vi "02 LinkTest.vi"(8 "error in (no error)":errorcluster caption="错误输入（无错误）", 10 "串口配置":T1={"VISA串口名称"="", "波特率"=9600, "停止位"=10, "流控制"=0, "数据位"=8, "奇偶校验"=enum."None", "超时"=2000, "启用终止符？"=FALSE, "终止符"=10} {"终止符" format="%.0x"; "数据位" min=5 max=8 step=1; "流控制" items=["无", "XON/XOFF", "RTS/CTS", "XON/XOFF & RTS/CTS", "DTR/DSR", "XON/XOFF & DTR/DSR"]; "停止位" items=["1.0"=10, "1.5"=15, "2.0"=20]; "波特率" items=["9600"=9600, "115200"=15]}, 11 "SerialClass 输入":refnum<class "SerialClass.lvclass">) -> (0 "error out":errorcluster caption="错误输出", 1 "串口已配置":T1={"VISA串口名称"="", "波特率"=9600, "停止位"=10, "流控制"=0, "数据位"=8, "奇偶校验"=enum."None", "超时"=2000, "启用终止符？"=FALSE, "终止符"=10} {"终止符" format="%.0x"; "数据位" min=5 max=8 step=1; "流控制" items=["无", "XON/XOFF", "RTS/CTS", "XON/XOFF & RTS/CTS", "DTR/DSR", "XON/XOFF & DTR/DSR"]; "停止位" items=["1.0"=10, "1.5"=15, "2.0"=20]; "波特率" items=["9600"=9600, "115200"=15]}, 2 "成功？":bool, 3 "SerialClass 输出":refnum<class "SerialClass.lvclass">)   [LabVIEW 2019, in "SerialClass.lvclass"]
uses:
  SerialClass.lvclass
  00 Ctl/SerialData.ctl
  <vilib>/Instr/_visa.llb/VISA Configure Serial Port (Instr).vi
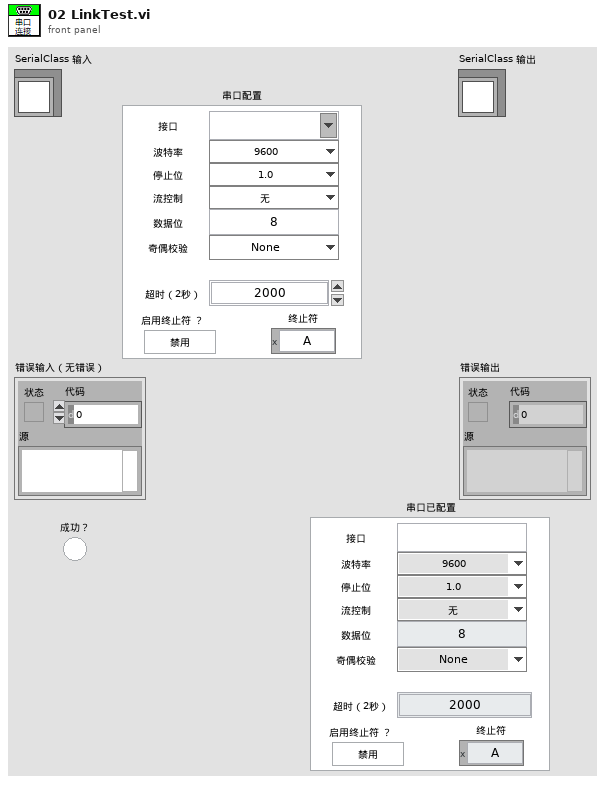
[diagram p1: front panel]
types:
  T1 = typedef "SerialData.ctl" = cluster{"VISA串口名称":refnum<visa-resource-name>, "波特率":u32, "停止位":u16, "流控制":u16, "数据位":u16, "奇偶校验":enum16{"None", "Odd", "Even", "Mark", "Space"}, "超时":u32, "启用终止符？":bool, "终止符":u8}
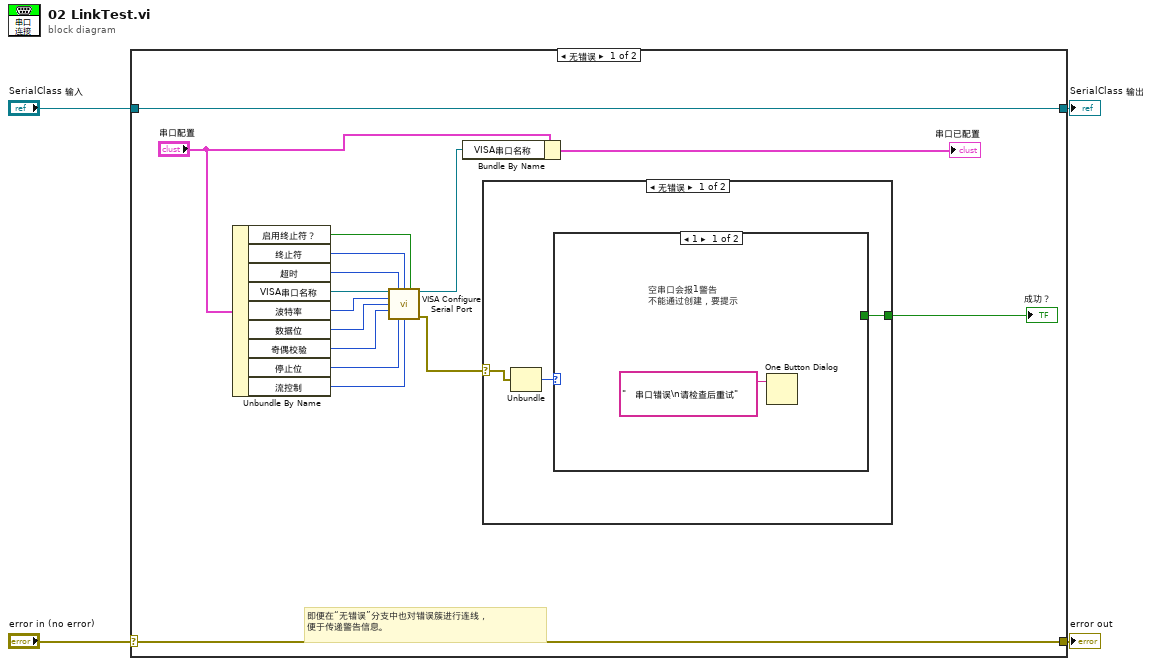
[diagram p0: block diagram]
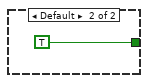
[diagram p2: hidden frame]
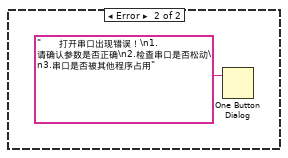
[diagram p3: hidden frame]
diagram:
  n1 = case shown="无错误" "error in (no error)" {
    selector: "error in (no error)" -> [w19 w28]
    tunnel: [w19 w28] -> w3
    tunnel: [w20 w27] -> w1
    tunnel: "SerialClass 输入" -> [w20 w27]
    frame No Error {
      # "即便在“无错误”分支中也对错误簇进行连线，\n便于传递警告信息。"
      n2 = Unbundle By Name("串口配置") -> ("启用终止符？"=w18:bool, "终止符"=w17:u8, "超时"=w16:u32, "VISA串口名称"=w15:refnum<visa-resource-name>, "波特率"=w14:u32, "数据位"=w13:u16, "奇偶校验"=w12:enum16{"None", "Odd", "Even", "Mark", "Space"}, "停止位"=w11:u16, "流控制"=w10:u16)
      n3 = call-poly "VISA Configure Serial Port"("VISA resource name"=w15, "timeout (10sec)"=w16, "termination char\n(0xA = '\\n' = LF)"=w17, "Enable Termination\nChar (T)"=w18, "baud rate (9600)"=w14, "data bits (8)"=w13, "parity (0:none)"=w12, "stop bits (10: 1 bit)"=w11, "flow control (0:none)"=w10) -> ("VISA resource name out"=w6:refnum<visa-resource-name>, "error out"=w9:errorcluster)  [unwired: 5 in]
      n4 = Bundle By Name(cluster="串口配置", "VISA串口名称"=w6) -> (→"串口已配置":T1)
      n5 = case shown="无错误" w9 {
        selector: w9 -> [w23 _]
        tunnel: [w21 _] -> w8
        frame No Error {
          n6 = Unbundle(w23) -> ("code"=w22:i32)  [unwired: 2 out]
          n7 = case shown="1" w22 {
            tunnel: [_ TRUE] -> w21
            frame 1 {
              # "空串口会报1警告\n不能通过创建，要提示"
              n8 = One Button Dialog(message="   串口错误\n请检查后重试" ("消息")) -> ()  [unwired: 1 in, 1 out]
            }
            frame Default {
            }
          }
        }
        frame Error {
          n9 = One Button Dialog(message="      打开串口出现错误！\n1.请确认参数是否正确\n2.检查串口是否松动\n3.串口是否被其他程序占用" ("消息")) -> ()  [unwired: 1 in, 1 out]
        }
      }
      "成功？" <- w8
    }
    frame Error {
    }
  }
  "error out" <- w3
  "SerialClass 输出" <- w1
